vi "Drive Controller.vi"(8 "error in":errorcluster) -> ()   [LabVIEW 2019]
doc: "This VI executes continuously carrying out the current operation and responding to updates or new operation requests. It will often contain the timing or control code that is difficult to place directly in TeleOp. This VI generally opens all sensors and motors and isolates the rest of the robot code from knowing implementation details of how the operations are carried out."
uses:
  <vilib>/Rock Robotics/WPI/Framework/Completion Status.ctl
  Drive Setpoints.ctl
  Drive Operations.ctl
  <vilib>/Rock Robotics/WPI/ThirdParty/REV Robotics/SPARK MAX/Typedef/Spark MAX Control Type.ctl
panel:
  in  "Interactive Values":T1
  in  "Buttons":cluster{"Execute Cmd":bool, "Abort Cmd":bool}
  out "Command Timing":cluster{"Start Time (ms)":u32, "Iterations":i32}
  out "Status":T3
  out "Setpoints":T4(graph)
  out "Current\nCmd":string
  # "Tip: The graph shows the motor setpoints. It may also be helpful to observe inputs and sensor values.\nYou may also want to display tuning or debugging controls."
  # "Interactive Command: You may fill in the settings for a command\nand schedule it with the Execute button. You can observe and abort\nany command while fine tuning the code for the controller."
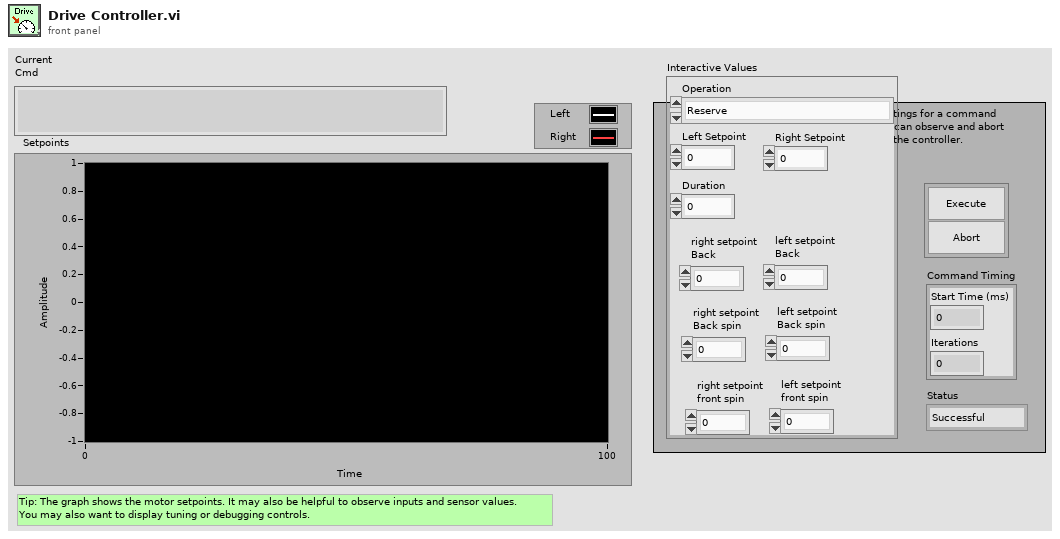
[diagram p1: front panel]
types:
  T1 = typedef "Drive Setpoints.ctl" = cluster{"Operation":T2, "Left Setpoint":dbl, "Right Setpoint":dbl, "Duration":dbl, "left setpoint\nBack":dbl, "right setpoint\nBack":dbl, "left setpoint\nBack spin":dbl, "right setpoint\nBack spin":dbl, "left setpoint \nfront spin":dbl, "right setpoint\nfront spin":dbl}
  T2 = typedef "Drive Operations.ctl" = enum16{"Reserve", "Read Current", "Immediate", "Drive for Time", "Drive for Distance"}
  T3 = typedef "Completion Status.ctl" = enum16{"Successful", "Aborted", "Incomplete"}
  T4 = cluster{"Left Setpoint":dbl, "Right Setpoint":dbl}
  T5 = typedef "WPI_MotorControlDeviceRef.ctl" = cluster{"DeviceStatus":errorcluster, "Type":T6, "PWM":cluster{"PWM Channel":T7, "DeadBand":T8}, "CAN":cluster{"Device Number":u8, "SetOutput VI Ref":variant, "GetOutput VI Ref":variant, "Enable VI Ref":variant, "Disable VI Ref":variant, "Data":variant}, "Invert":bool, "DIO PWM":cluster{"PWM \"Enable\" Channel":T7, "DIOChannel":T9, "PWM Rate":dbl}}
  T6 = typedef "WPI_MotorControlType.ctl" = enum16{"PWM", "CAN", "DIO PWM"}
  T7 = typedef "FPGA_DIOPWMChannel.ctl" = enum8{"PWM 0", "PWM 1", "PWM 2", "PWM 3", "PWM 4", "PWM 5", "PWM 6", "PWM 7", "PWM 8", "PWM 9", "PWM MXP 0", "PWM MXP 1", "PWM MXP 2", "PWM MXP 3", "PWM MXP 4", "PWM MXP 5", "PWM MXP 6", "PWM MXP 7", "PWM MXP 8", "PWM MXP 9", "Invalid"}
  T8 = typedef "WPI_PWMDeadband.ctl" = cluster{"Name":string, "maxPositivePwm":i32, "minPositivePwm":i32, "centerPwm":i32, "maxNegativePwm":i32, "minNegativePwm":i32, "angularRange":u16}
  T9 = typedef "FPGA_DIOChannel.ctl" = enum8{"DIO 0", "DIO 1", "DIO 2", "DIO 3", "DIO 4", "DIO 5", "DIO 6", "DIO 7", "DIO 8", "DIO 9", "DIO MXP 0", "DIO MXP 1", "DIO MXP 2", "DIO MXP 3", "DIO MXP 4", "DIO MXP 5", "DIO MXP 6", "DIO MXP 7", "DIO MXP 8", "DIO MXP 9", "DIO MXP 10", "DIO MXP 11", "DIO MXP 12", "DIO MXP 13", "DIO MXP 14", "DIO MXP 15", "SPI Port CS1", "SPI Port CS2", "SPI Port CS3", "SPI Port MISO", "SPI Port MOSI", "Invalid"}
  T10 = cluster{"error out":errorcluster, "error out":errorcluster, "error out":errorcluster, "error out":errorcluster}
  T11 = cluster{"MotorControlDeviceRef":T5, "MotorControlDeviceRef":T5, "MotorControlDeviceRef":T5, "MotorControlDeviceRef":T5, "error out":errorcluster, "error out":errorcluster, "error out":errorcluster, "error out":errorcluster}
  T12 = typedef "Command Status Info.ctl" = cluster{"Name":string, "Status":T3, "notifier out":T13}
  T13 = typedef "Completion Notifier.ctl" = refnum<notifier>
  T14 = cluster{"SubSystem Data":T1, cluster{"Start Time (ms)":u32, "Iterations":i32}, cluster{"Command Info":T12, "Description":string, "Default Command":T1, "queue out":refnum<queue>, "Subsystem Name":string}}
  T15 = typedef "Spark MAX Control Type.ctl" = enum16{"Percent VBus", "Voltage", "Velocity", "Position", "Smart Motion", "Current", "Smart Velocity"}
  T16 = cluster{"left setpoint\nBack spin":dbl, "right setpoint\nBack spin":dbl, "left setpoint \nfront spin":dbl, "right setpoint\nfront spin":dbl}
  T17 = cluster{"Don't move motors while reserved":dbl, "Don't move motors while reserved":dbl, "Don't move motors while reserved":dbl, "Don't move motors while reserved":dbl}
  T18 = cluster{"Don't move motors while reserved":dbl, "Don't move motors while reserved":dbl}
  T19 = cluster{"SubSystem Data":T1, cluster{"Start Time (ms)":u32, "Iterations":i32}, "Default Command Arguments":cluster{"Command Info":T12, "Description":string, "Default Command":T1, "queue out":refnum<queue>, "Subsystem Name":string}}
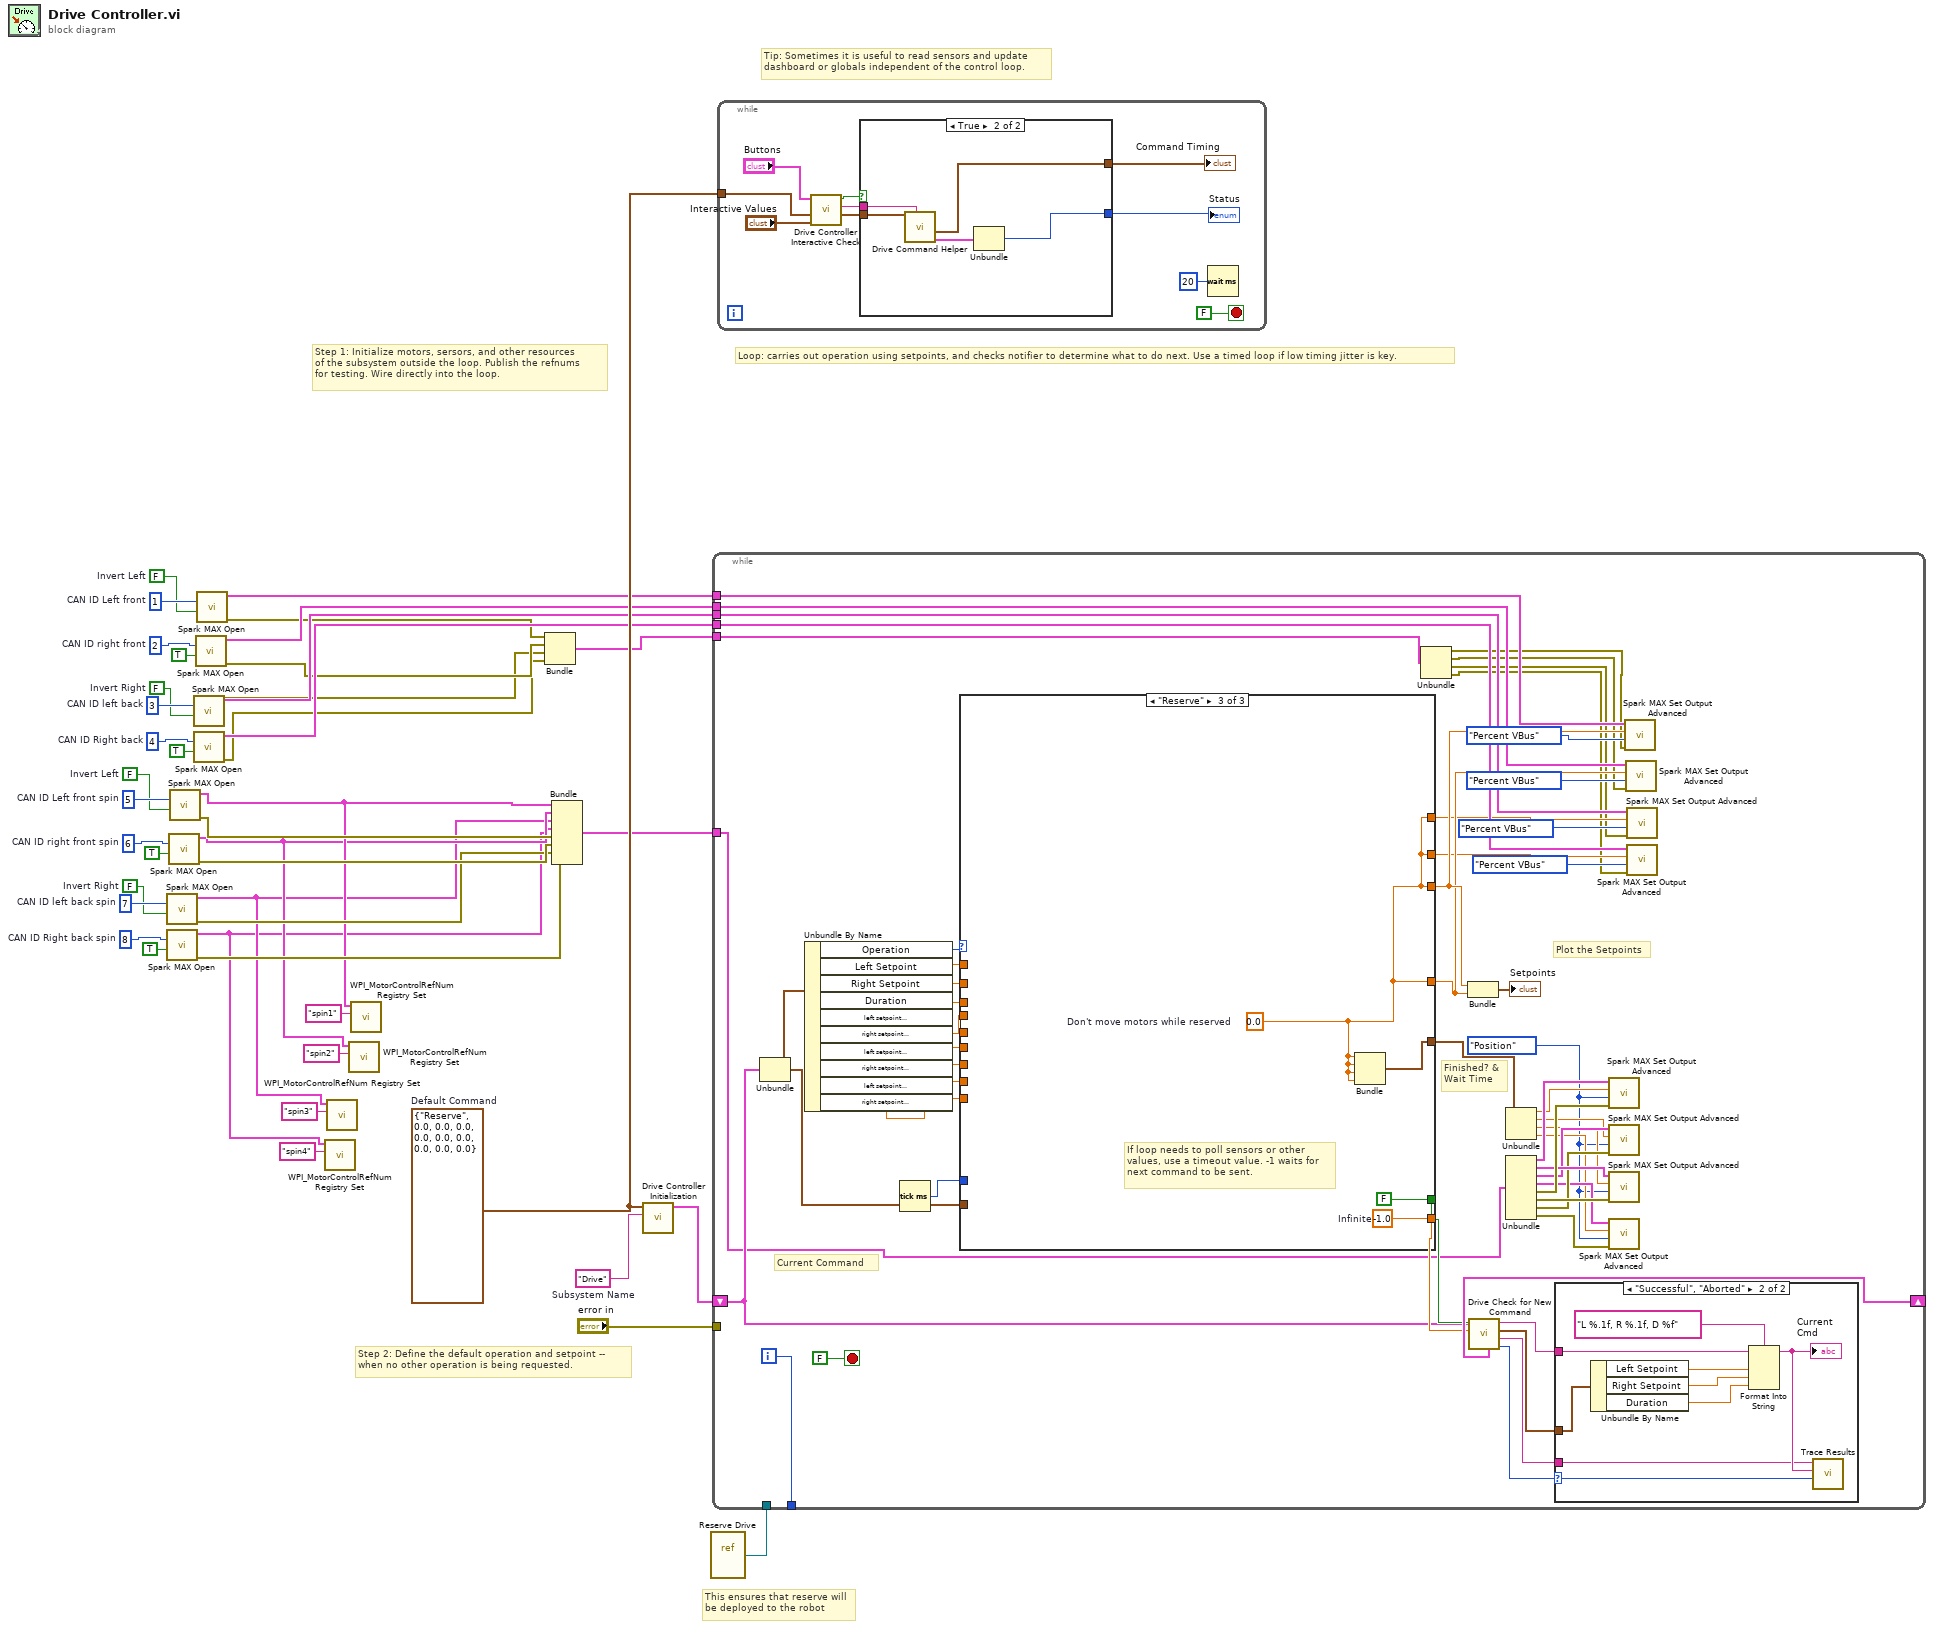
[diagram p0: block diagram]
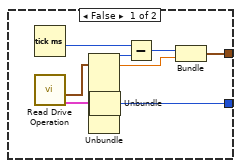
[diagram p2: hidden frame]
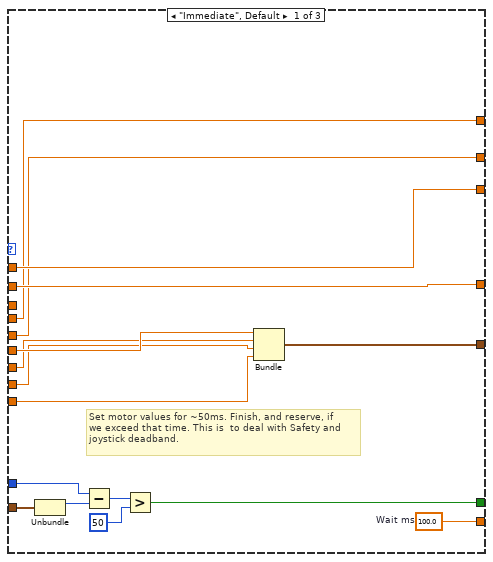
[diagram p4: hidden frame]
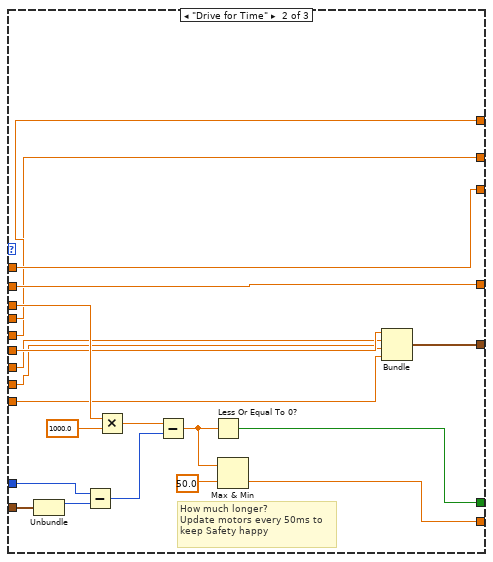
[diagram p5: hidden frame]
diagram:
  w15 = FALSE  # Invert Left
  w16 = FALSE  # Invert Right
  w18 = u8 7  # CAN ID left back spin
  w17 = u8 8  # CAN ID Right back spin
  w19 = u8 5  # CAN ID Left front spin
  w20 = u8 6  # CAN ID right front spin
  w33 = FALSE  # Invert Left
  w34 = FALSE  # Invert Right
  w36 = u8 3  # CAN ID left back
  w35 = u8 4  # CAN ID Right back
  w37 = u8 1  # CAN ID Left front
  w38 = u8 2  # CAN ID right front
  w39 = T1 {"Operation"=enum."Reserve", "Left Setpoint"=0.0, "Right Setpoint"=0.0, "Duration"=0.0, "left setpoint\nBack"=0.0, "right setpoint\nBack"=0.0, "left setpoint\nBack spin"=0.0, "right setpoint\nBack spin"=0.0, "left setpoint \nfront spin"=0.0, "right setpoint\nfront spin"=0.0}  # Default Command
  w43 = "Drive"  # Subsystem Name
  # "This ensures that reserve will\nbe deployed to the robot"
  # "Tip: Sometimes it is useful to read sensors and update\ndashboard or globals independent of the control loop."
  # "Step 2: Define the default operation and setpoint --\nwhen no other operation is being requested."
  # "Step 1: Initialize motors, sersors, and other resources\nof the subsystem outside the loop. Publish the refnums\nfor testing. Wire directly into the loop."
  # "Loop: carries out operation using setpoints, and checks notifier to determine what to do next. Use a timed loop if low timing jitter is key."
  n1 = call <vilib>:"Spark MAX Open.vi"("Invert"=w16, "Device Number"=w18) -> ("error out"=w10:errorcluster, "MotorControlDeviceRef"=w2:T5)  [unwired: 8 in]
  n2 = call <vilib>:"Spark MAX Open.vi"("Invert"=TRUE, "Device Number"=w17) -> ("error out"=w9:errorcluster, "MotorControlDeviceRef"=w1:T5)  [unwired: 8 in]
  n3 = call <vilib>:"Spark MAX Open.vi"("Invert"=TRUE, "Device Number"=w20) -> ("error out"=w11:errorcluster, "MotorControlDeviceRef"=w5:T5)  [unwired: 8 in]
  n4 = call <vilib>:"Spark MAX Open.vi"("Invert"=w15, "Device Number"=w19) -> ("error out"=w12:errorcluster, "MotorControlDeviceRef"=w8:T5)  [unwired: 8 in]
  n5 = call <vilib>:"Spark MAX Open.vi"("Invert"=w34, "Device Number"=w36) -> ("error out"=w26:errorcluster, "MotorControlDeviceRef"=w30:T5)  [unwired: 8 in]
  n6 = call <vilib>:"Spark MAX Open.vi"("Invert"=TRUE, "Device Number"=w35) -> ("error out"=w25:errorcluster, "MotorControlDeviceRef"=w29:T5)  [unwired: 8 in]
  n7 = call <vilib>:"Spark MAX Open.vi"("Invert"=TRUE, "Device Number"=w38) -> ("error out"=w27:errorcluster, "MotorControlDeviceRef"=w31:T5)  [unwired: 8 in]
  n8 = call <vilib>:"Spark MAX Open.vi"("Invert"=w33, "Device Number"=w37) -> ("error out"=w28:errorcluster, "MotorControlDeviceRef"=w32:T5)  [unwired: 8 in]
  n9 = call <vilib>:"WPI_MotorControlRefNum Registry Set.vi"("refnum name"="spin4", "MotorControlDevRef"=w1) -> ()  [unwired: 8 in, 2 out]
  n10 = call <vilib>:"WPI_MotorControlRefNum Registry Set.vi"("refnum name"="spin3", "MotorControlDevRef"=w2) -> ()  [unwired: 8 in, 2 out]
  n11 = call <vilib>:"WPI_MotorControlRefNum Registry Set.vi"("refnum name"="spin2", "MotorControlDevRef"=w5) -> ()  [unwired: 8 in, 2 out]
  n12 = call <vilib>:"WPI_MotorControlRefNum Registry Set.vi"("refnum name"="spin1", "MotorControlDevRef"=w8) -> ()  [unwired: 8 in, 2 out]
  n13 = Bundle("error out"=w28, "error out"=w27, "error out"=w26, "error out"=w25) -> (w24:T10)  [unwired: 1 in]
  n14 = Bundle("MotorControlDeviceRef"=w8, "MotorControlDeviceRef"=w5, "MotorControlDeviceRef"=w2, "MotorControlDeviceRef"=w1, "error out"=w12, "error out"=w11, "error out"=w10, "error out"=w9) -> (w21:T11)  [unwired: 1 in]
  n15 = call "Drive Controller Initialization.vi"("Subsystem Name"=w43, "Default Command"=w39) -> ("Current Command"=w41:T14)  [unwired: 9 in]
  n16 = vi-ref "Reserve Drive.vi"() -> (w40:refnum<vi>)
  n17 = while {
    shift-right: [w89] -> _
    shift-left: w41 -> [w82]
    tunnel: [w98] -> _
    tunnel: "error in" -> [_]
    tunnel: w40 -> [_]
    tunnel: w32 -> [w75]
    tunnel: w31 -> [w74]
    tunnel: w30 -> [w73]
    tunnel: w29 -> [w72]
    tunnel: w24 -> [w63]
    tunnel: w21 -> [w58]
    i -> [w98]
    stop <- FALSE stop-if-true
    w44 = Spark_MAX_Control_Type."Position" ("Control Mode")
    # "Current Command"
    # "Plot the Setpoints"
    # "Finished? &\nWait Time"
    n18 = Unbundle(w82) -> ("SubSystem Data"=w96:T1, w83:cluster{"Start Time (ms)":u32, "Iterations":i32})  [unwired: 1 out]
    n19 = Unbundle By Name(w96) -> ("Operation"=w95:T2, "Left Setpoint"=w94:dbl, "Right Setpoint"=w93:dbl, "Duration"=w92:dbl, "left setpoint\nBack"=w81:dbl, "right setpoint\nBack"=w80:dbl, "left setpoint\nBack spin"=w79:dbl, "right setpoint\nBack spin"=w78:dbl, "left setpoint \nfront spin"=w77:dbl, "right setpoint\nfront spin"=w76:dbl)
    n20 = Tick Count (ms)() -> (millisecond timer value=w91:u32)
    n21 = case shown="\"Reserve\"" w95 {
      tunnel: [w124 w132 w148] -> w88
      tunnel: [w117 w139 FALSE ("ignore previous (F)")] -> w87
      tunnel: w83 -> [w116 w141 _]
      tunnel: [w123 w138 w146] -> w71
      tunnel: [w122 w137 w146] -> w70
      tunnel: w94 -> [w123 w138 _]
      tunnel: w93 -> [w122 w137 _]
      tunnel: w92 -> [_ w136 _]
      tunnel: w91 -> [w118 w135 _]
      tunnel: w81 -> [w115 w131 _]
      tunnel: w80 -> [w114 w130 _]
      tunnel: w79 -> [w113 w128 _]
      tunnel: w78 -> [w112 w127 _]
      tunnel: w77 -> [w111 w126 _]
      tunnel: w76 -> [w110 w125 _]
      tunnel: [w115 w131 w146] -> w69
      tunnel: [w114 w130 w146] -> w68
      tunnel: [w109 w129 w145] -> w57
      frame "Immediate", Default {
        w124 = 100.0  # Wait ms
        # "Set motor values for ~50ms. Finish, and reserve, if\nwe exceed that time. This is  to deal with Safety and\njoystick deadband."
        n22 = Unbundle(w116) -> ("Start Time (ms)"=w119:u32)  [unwired: 1 out]
        n23 = Subtract(x=w118, y=w119) -> (x-y=w120:u32)
        n24 = Greater?(x=w120, y=u8 50 ("Left Motor")) -> (0:w117:bool)
        n25 = Bundle("left setpoint\nBack spin"=w113, "right setpoint\nBack spin"=w112, "left setpoint \nfront spin"=w111, "right setpoint\nfront spin"=w110) -> (w109:T16)  [unwired: 1 in]
      }
      frame "Drive for Time" {
        # "How much longer?\nUpdate motors every 50ms to\nkeep Safety happy"
        n26 = Unbundle(w141) -> ("Start Time (ms)"=w140:u32)  [unwired: 1 out]
        n27 = Subtract(x=w135, y=w140) -> (x-y=w144:u32)
        n28 = Multiply(x=w136, y=1000.0) -> (x*y=w143:dbl)
        n29 = Subtract(x=w143, y=w144) -> (x-y=w134:dbl)
        n30 = Less Or Equal To 0?(x=w134) -> (x <= 0?=w139:bool)
        n31 = Max & Min(x=w134, y=50.0) -> (min(x,y)=w132:dbl)  [unwired: 1 out]
        n32 = Bundle("left setpoint\nBack spin"=w128, "right setpoint\nBack spin"=w127, "left setpoint \nfront spin"=w126, "right setpoint\nfront spin"=w125) -> (w129:T16)  [unwired: 1 in]
      }
      frame "Reserve" {
        w146 = 0.0  # Don't move motors while reserved
        w148 = -1.0  # Infinite
        # "If loop needs to poll sensors or other\nvalues, use a timeout value. -1 waits for\nnext command to be sent."
        n33 = Bundle("Don't move motors while reserved"=w146, "Don't move motors while reserved"=w146, "Don't move motors while reserved"=w146, "Don't move motors while reserved"=w146) -> (w145:T17)  [unwired: 1 in]
      }
    }
    n34 = Unbundle(w63) -> ("error out"=w62:errorcluster, "error out"=w61:errorcluster, "error out"=w60:errorcluster, "error out"=w59:errorcluster)
    n35 = Bundle("Don't move motors while reserved"=w71, "Don't move motors while reserved"=w70) -> (→"Setpoints":T18)  [unwired: 1 in]
    n36 = call "Drive Check for New Command.vi"("input cluster"=w82, "Wait time (ms)"=w88, "Finished?"=w87) -> ("Completion"=w90:T3, "Subsystem Name"=w84:string, "Current Command"=w85:T1, "Initial Trace String"=w86:string, "Next Command"=w89:T19)  [unwired: 4 in]
    n37 = Unbundle(w57) -> ("Don't move motors while reserved"=w48:dbl, "Don't move motors while reserved"=w47:dbl, "Don't move motors while reserved"=w46:dbl, "Don't move motors while reserved"=w45:dbl)
    n38 = Unbundle(w58) -> ("MotorControlDeviceRef"=w56:T5, "MotorControlDeviceRef"=w54:T5, "MotorControlDeviceRef"=w52:T5, "MotorControlDeviceRef"=w50:T5, "error out"=w55:errorcluster, "error out"=w53:errorcluster, "error out"=w51:errorcluster, "error out"=w49:errorcluster)
    n39 = case shown="\"Successful\", \"Aborted\"" w90 {
      selector: w90 -> [_ w108]
      tunnel: w86 -> [_ w103]
      tunnel: w85 -> [_ w104]
      tunnel: w84 -> [_ w100]
      frame "Incomplete", Default {
        # "Continuing current command"
      }
      frame "Successful", "Aborted" {
        # "Report and setup for next command"
        n40 = Unbundle By Name(w104) -> ("Left Setpoint"=w106:dbl, "Right Setpoint"=w107:dbl, "Duration"=w101:dbl)
        n41 = Format Into String(format string="L %.1f, R %.1f, D %f", initial string=w103, w106, w107, w101) -> (resulting string=w102:string)  [unwired: 1 in, 1 out]
        "Current\nCmd" <- w102
        n42 = call <vilib>:"Trace Results.vi"("Status of previous command"=w108, "Description"=w102, "Subsystem"=w100) -> ()  [unwired: 9 in]
      }
    }
    n43 = call <vilib>:"Spark MAX Set Output Advanced.vi"("error in (no error)"=w55, "Control Mode"=w44, "Setpoint"=w48, "MotorControlDevRef"=w56) -> ()  [unwired: 6 in, 2 out]
    n44 = call <vilib>:"Spark MAX Set Output Advanced.vi"("error in (no error)"=w51, "Control Mode"=w44, "Setpoint"=w47, "MotorControlDevRef"=w52) -> ()  [unwired: 6 in, 2 out]
    n45 = call <vilib>:"Spark MAX Set Output Advanced.vi"("error in (no error)"=w53, "Control Mode"=w44, "Setpoint"=w46, "MotorControlDevRef"=w54) -> ()  [unwired: 6 in, 2 out]
    n46 = call <vilib>:"Spark MAX Set Output Advanced.vi"("error in (no error)"=w49, "Control Mode"=w44, "Setpoint"=w45, "MotorControlDevRef"=w50) -> ()  [unwired: 6 in, 2 out]
    n47 = call <vilib>:"Spark MAX Set Output Advanced.vi"("error in (no error)"=w62, "Control Mode"=Spark_MAX_Control_Type."Percent VBus", "Setpoint"=w71, "MotorControlDevRef"=w75) -> ()  [unwired: 6 in, 2 out]
    n48 = call <vilib>:"Spark MAX Set Output Advanced.vi"("error in (no error)"=w61, "Control Mode"=Spark_MAX_Control_Type."Percent VBus", "Setpoint"=w70, "MotorControlDevRef"=w74) -> ()  [unwired: 6 in, 2 out]
    n49 = call <vilib>:"Spark MAX Set Output Advanced.vi"("error in (no error)"=w60, "Control Mode"=Spark_MAX_Control_Type."Percent VBus", "Setpoint"=w69, "MotorControlDevRef"=w73) -> ()  [unwired: 6 in, 2 out]
    n50 = call <vilib>:"Spark MAX Set Output Advanced.vi"("error in (no error)"=w59, "Control Mode"=Spark_MAX_Control_Type."Percent VBus", "Setpoint"=w68, "MotorControlDevRef"=w72) -> ()  [unwired: 6 in, 2 out]
  }
  n51 = while {
    tunnel: w39 -> [w150]
    stop <- FALSE stop-if-true
    n52 = call "Drive Controller Interactive Check.vi"("Interactive Command In"="Interactive Values", "Default Command"=w150, "Buttons"="Buttons") -> ("Interactive Command Out"=w152:T1, "Trace String"=w153:string, "Schedule"=w154:bool)  [unwired: 6 in]
    n53 = case shown="True" w154 {
      tunnel: [w163 w171] -> w155
      tunnel: [w162 w167] -> w156
      tunnel: w153 -> [_ w169]
      tunnel: w152 -> [_ w168]
      frame False {
        n54 = Tick Count (ms)() -> (millisecond timer value=w166:u32)
        n55 = call "Read Drive Operation.vi"() -> ("Command Info"=w160:T12, "SubSystem Data"=w159:T1)  [unwired: 9 in, 1 out]
        n56 = Unbundle(w159) -> ("Operation"=w164:T2, "Left Setpoint"=w161:dbl)  [unwired: 8 out]
        n57 = Unbundle(w160) -> ("Status"=w163:T3)  [unwired: 2 out]
        n58 = Subtract(x=w166, y=w164) -> (x-y=w165:u32)
        n59 = Bundle(w165, "Left Setpoint"=w161) -> (w162:cluster{u32, "Left Setpoint":dbl})  [unwired: 1 in]
      }
      frame True {
        n60 = call "Drive Command Helper.vi"("Description"=w169, "SubSystem Data"=w168) -> ("Command Info Out"=w170:T12, "Command Timing"=w167:cluster{"Start Time (ms)":u32, "Iterations":i32})  [unwired: 7 in, 1 out]
        n61 = Unbundle(w170) -> ("Status"=w171:T3)  [unwired: 2 out]
      }
    }
    "Status" <- w155
    "Command Timing" <- w156
    n62 = Wait (ms)(milliseconds to wait=u32 20) -> ()  [unwired: 1 out]
  }
